vi "Manage ROI.vi"(3 "Switch X/Y":bool, 4 "Trap cluster in":T2, 5 "ROI in":T1, 6 "Group traps":bool) -> (0 "Replace ROI":bool, 1 "ROI out":T1, 2 "Previous ROI out":T1)   [LabVIEW 2011]
uses:
  Trap cluster.ctl
panel:
  in  "Handle":T1={"Global Rectangle"=[254, 259, 368, 261], "Contours"=[{"Contour Type"=0, "ROI Type"=2, "Points"=[254, 260, 367, 259]}]}
  out "Temp ROI":T1
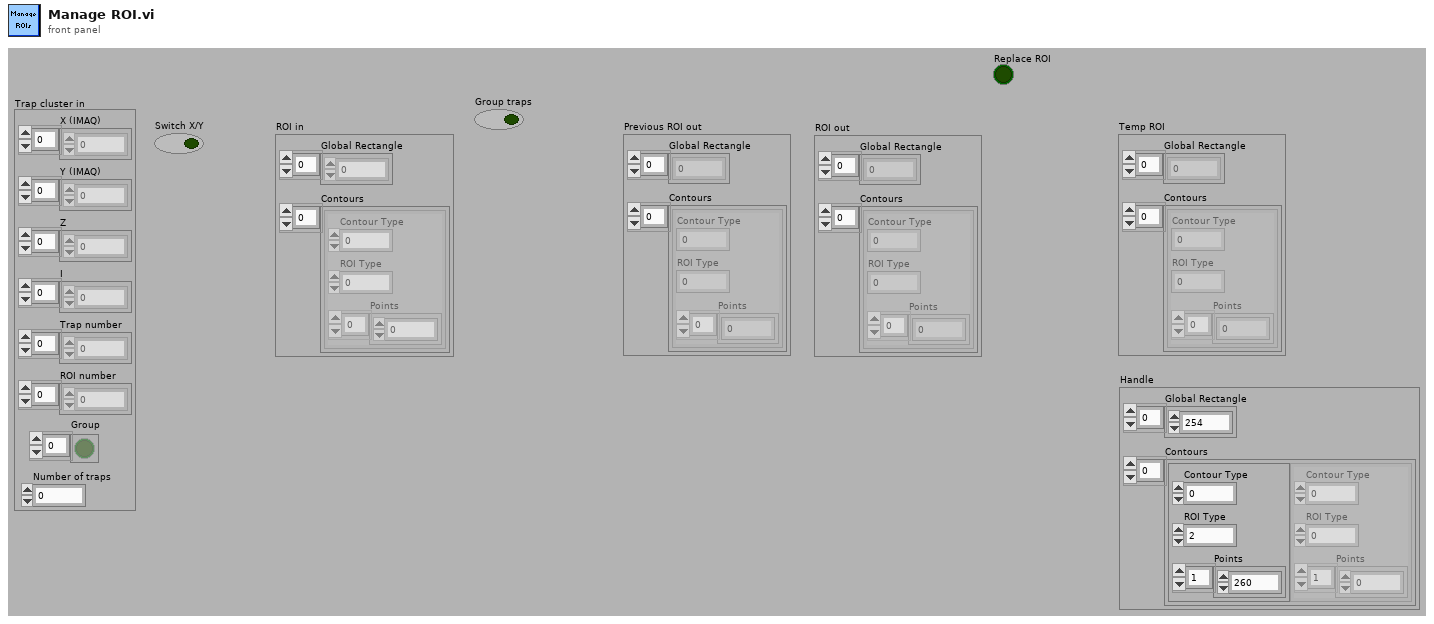
[diagram p1: front panel]
types:
  T1 = cluster{"Global Rectangle":i32[], "Contours":cluster{"Contour Type":u32, "ROI Type":u32, "Points":i32[]}[]}
  T2 = typedef "Trap cluster.ctl" = cluster{"X (IMAQ)":sgl[], "Y (IMAQ)":sgl[], "Z":sgl[], "I":sgl[], "Trap number":i32[], "ROI number":i32[], "Number of traps":i32, "Group":bool[]}
  T3 = cluster{"Contour Type":u32, "ROI Type":u32, "Points":i32[]}[]
  T4 = cluster{"Contour Type":u32, "ROI Type":u32, "Points":i32[]}
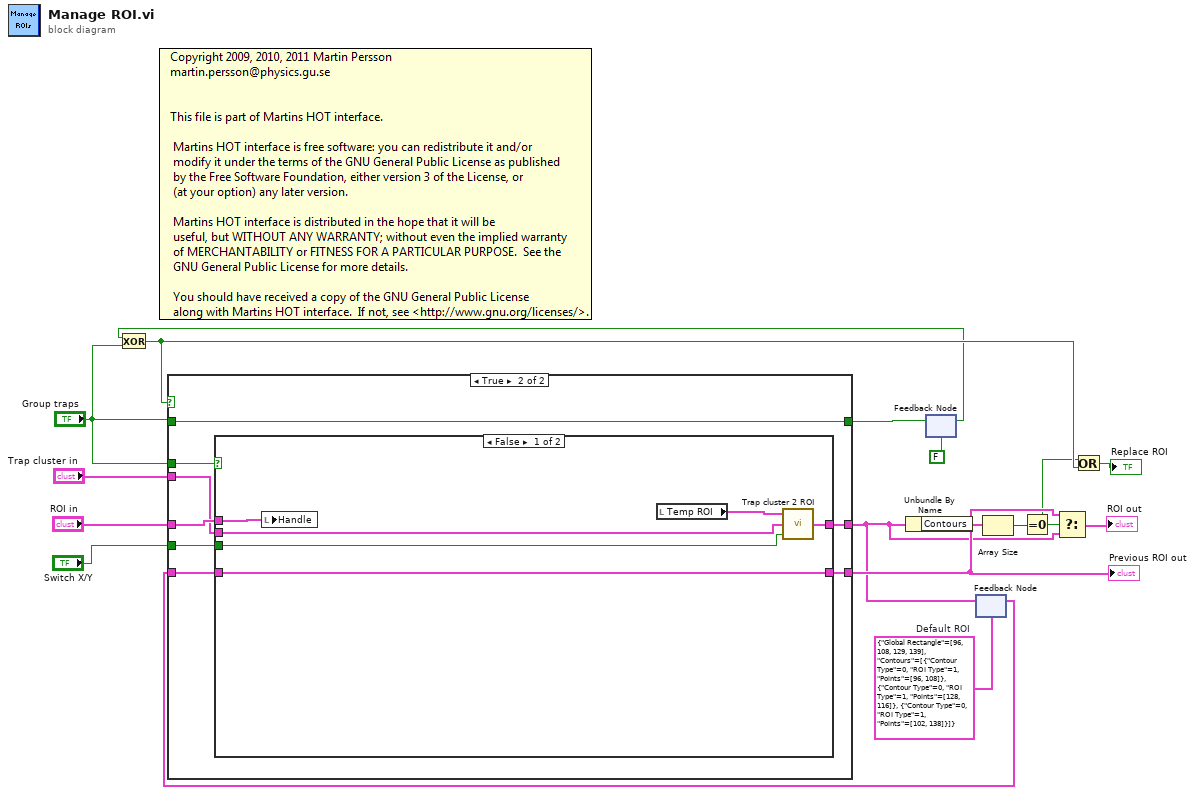
[diagram p0: block diagram]
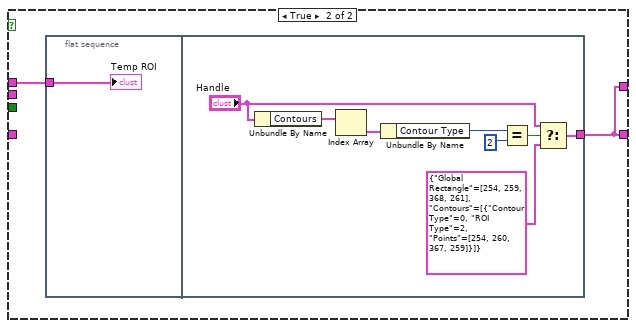
[diagram p3: hidden frame]
diagram:
  w1 = T1 {"Global Rectangle"=[96, 108, 129, 139], "Contours"=[{"Contour Type"=0, "ROI Type"=1, "Points"=[96, 108]}, {"Contour Type"=0, "ROI Type"=1, "Points"=[128, 116]}, {"Contour Type"=0, "ROI Type"=1, "Points"=[102, 138]}]}  # Default ROI
  n1 = feedback #1(FALSE ("Group traps")) -> (w13:bool)
  n2 = Exclusive Or(1:"Group traps", 2:w13) -> (0:w16:bool)
  n3 = feedback #2(w1) -> (w11:T1)
  n4 = case shown="True" w16 {
    tunnel: "Group traps" -> [_ w28]
    tunnel: "ROI in" -> [w20 w26]
    tunnel: [w20 w27] -> w5
    tunnel: w11 -> [w19 w25]
    tunnel: [w19 w24] -> w6
    tunnel: "Trap cluster in" -> [_ w23]
    tunnel: "Group traps" -> [w18 w22]
    tunnel: [w18 w22] -> w14
    tunnel: "Switch X/Y" -> [_ w21]
    frame False {
    }
    frame True {
      n5 = case shown="False" w28 {
        tunnel: w26 -> [w30 w36]
        tunnel: [w33 w35] -> w27
        tunnel: w25 -> [w34 _]
        tunnel: [w34 w35] -> w24
        tunnel: w23 -> [w32 _]
        tunnel: w21 -> [w29 _]
        frame False {
          n6 = local write "Handle"(w30) -> ()
          n7 = local read "Temp ROI"() -> (w31:T1)
          n8 = call "Trap cluster 2 ROI.vi"("Switch X/Y"=w29, "Trap cluster"=w32, "ROI in"=w31) -> ("ROI out"=w33:T1)
        }
        frame True {
          n9 = flat-sequence {
            tunnel: w36 -> [w37]
            tunnel: [w38] -> w35
            frame #0 {
              "Temp ROI" <- w37
            }
            frame #1 {
              n10 = Unbundle By Name("Handle") -> ("Contours"=w45:T3)
              n11 = Index Array(array=w45) -> (element=w44:T4)  [unwired: 1 in]
              n12 = Unbundle By Name(w44) -> ("Contour Type"=w43:u32)
              n13 = Equal?(x=w43, y=u32 2) -> (x = y?=w41:bool)
              n14 = Select(t="Handle", s=w41, f=T1 {"Global Rectangle"=[254, 259, 368, 261], "Contours"=[{"Contour Type"=0, "ROI Type"=2, "Points"=[254, 260, 367, 259]}]} ("ROI")) -> (s? t:f=w38:T1)
            }
          }
        }
      }
    }
  }
  "Previous ROI out" <- w6
  n15 = Unbundle By Name(w5) -> ("Contours"=w8:T3)
  n16 = feedback-in #1(w14) -> ()
  n17 = feedback-in #2(w5) -> ()
  n18 = Array Size(array=w8) -> (size(s)=w7:i32)
  n19 = Equal To 0?(x=w7) -> (x = 0?=w2:bool)
  n20 = Select(t=w6, s=w2, f=w5) -> (s? t:f=→"ROI out":T1)
  n21 = Or(x=w2, y=w16) -> (x .or. y?=→"Replace ROI":bool)
